vi "Recall Data From File.vi"(4 "Waveform Generator (0: Waveform Generator 1)":i32(ring) items=["Waveform Generator 1", "Waveform Generator 2"], 5 "Serial Bus Name (1: Serial Bus 1)":i32(ring)=1 items=["Serial Bus 1"=1, "Serial Bus 2"=2], 6 "Arbitrary column Number (1)":i32=1, 7 "Internal Location":string, 8 "error in (no error)":errorcluster, 9 "Waveform Memory Location (1: Waveform Memory 1)":i32(ring)=1 items=["Waveform Memory 1"=1, "Waveform Memory 2"=2], 10 "File Type (0: Mask)":i32(ring) items=["Mask", "Setup", "Waveform", "Arbitrary", "DBC", "LDF"], 11 "VISA resource name":refnum<visa-resource-name>) -> (0 "error out":errorcluster, 3 "VISA resource name out":refnum<visa-resource-name>)   [LabVIEW 2015, in "Agilent 2000 3000 X-Series.lvlib"]
doc: "Configure the recall file operation."
uses:
  <instrlib>/Agilent 2000 3000 X-Series/Agilent 2000 3000 X-Series.lvlib
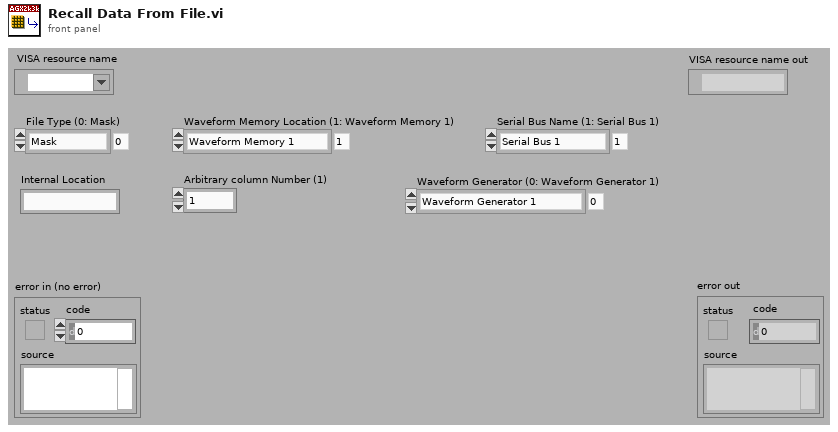
[diagram p1: front panel]
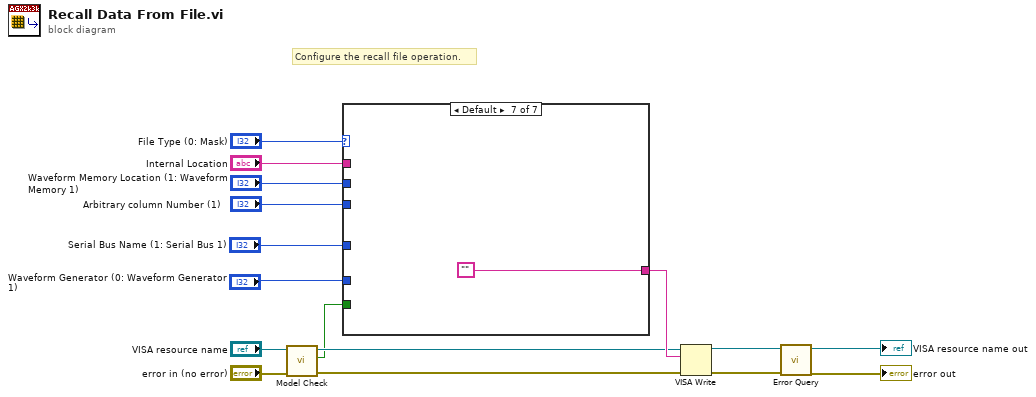
[diagram p0: block diagram]
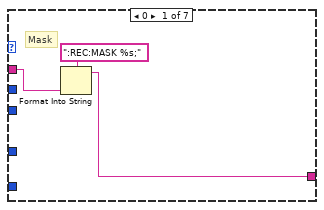
[diagram p2: hidden frame]
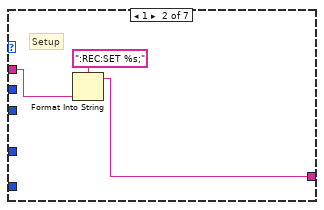
[diagram p3: hidden frame]
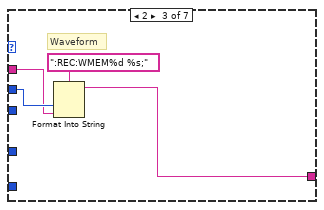
[diagram p4: hidden frame]
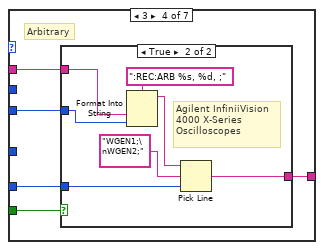
[diagram p5: hidden frame]
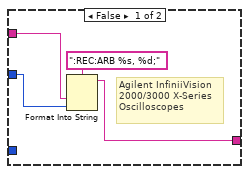
[diagram p6: hidden frame]
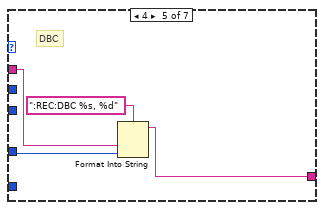
[diagram p7: hidden frame]
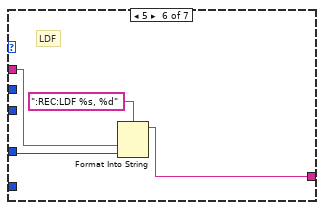
[diagram p8: hidden frame]
diagram:
  # "Configure the recall file operation."
  n1 = call <instrlib>:"Model Check.vi"("error in (no error)"="error in (no error)", "VISA resource name"="VISA resource name") -> ("error out"=w3:errorcluster, "Not 2000 or 3000 Series"=w2:bool, "VISA resource name out"=w4:refnum<visa-resource-name>)  [unwired: 7 out]
  n2 = case shown="Default" "File Type (0: Mask)" {
    tunnel: "Internal Location" -> [w19 w21 w24 w31 w46 w50 _]
    tunnel: "Waveform Memory Location (1: Waveform Memory 1)" -> [_ _ w25 _ _ _ _]
    tunnel: [w17 w20 w23 w29 w44 w48 ""] -> w9
    tunnel: "Arbitrary column Number (1)" -> [_ _ _ w30 _ _ _]
    tunnel: "Waveform Generator (0: Waveform Generator 1)" -> [_ _ _ w28 _ _ _]
    tunnel: w2 -> [_ _ _ w27 _ _ _]
    tunnel: "Serial Bus Name (1: Serial Bus 1)" -> [_ _ _ _ w45 w49 _]
    frame 0 {
      # "Mask"
      n3 = Format Into String(format string=":REC:MASK %s;", w19) -> (resulting string=w17:string)  [unwired: 2 in, 1 out]
    }
    frame 1 {
      # "Setup"
      n4 = Format Into String(format string=":REC:SET %s;", w21) -> (resulting string=w20:string)  [unwired: 2 in, 1 out]
    }
    frame 2 {
      # "Waveform"
      n5 = Format Into String(format string=":REC:WMEM%d %s;", w25, w24) -> (resulting string=w23:string)  [unwired: 2 in, 1 out]
    }
    frame 3 {
      # "Arbitrary"
      n6 = case shown="True" w27 {
        tunnel: w31 -> [w35 w41]
        tunnel: w30 -> [w34 w40]
        tunnel: [w33 w36] -> w29
        tunnel: w28 -> [_ w37]
        frame False {
          # "Agilent InfiniiVision\n2000/3000 X-Series\nOscilloscopes"
          n7 = Format Into String(format string=":REC:ARB %s, %d;", w35, w34) -> (resulting string=w33:string)  [unwired: 2 in, 1 out]
        }
        frame True {
          # "Agilent InfiniiVision\n4000 X-Series\nOscilloscopes"
          n8 = Format Into String(format string=":REC:ARB %s, %d, ;", w41, w40) -> (resulting string=w39:string)  [unwired: 2 in, 1 out]
          n9 = Pick Line(string ("")=w39, multi-line string="WGEN1;\nWGEN2;", line index=w37) -> (output string=w36:string)
        }
      }
    }
    frame 4 {
      # "DBC"
      n10 = Format Into String(format string=":REC:DBC %s, %d", w46, w45) -> (resulting string=w44:string)  [unwired: 2 in, 1 out]
    }
    frame 5 {
      # "LDF"
      n11 = Format Into String(format string=":REC:LDF %s, %d", w50, w49) -> (resulting string=w48:string)  [unwired: 2 in, 1 out]
    }
    frame Default {
    }
  }
  n12 = VISA Write(VISA resource name=w4, write buffer=w9, error in (no error)=w3) -> (VISA resource name out=w16:refnum<visa-resource-name>, error out=w15:errorcluster)  [unwired: 1 out]
  n13 = call <instrlib>:"Error Query.vi"("error in (no error)"=w15, "VISA resource name"=w16) -> ("error out"=→"error out":errorcluster, "VISA resource name out"=→"VISA resource name out":refnum<visa-resource-name>)  [unwired: 8 out]
